vi "PostBuild.vi"(8 "error in (no error)":errorcluster, 9 "GeneratedFiles in":path[](array[path]), 10 "GeneratedDirectories in":path[](array[path]), 11 "Class in":refnum<class "Installer.lvclass">) -> (0 "error out":errorcluster, 1 "GeneratedFiles out":path[](array[path]), 2 "GeneratedDirectories out":path[](array[path]), 3 "Class out":refnum<class "Installer.lvclass">)   [LabVIEW 2020, in "Installer.lvclass"]
uses:
  <vilib>/AppBuilder/IB_Classes/Installer/Installer.lvclass
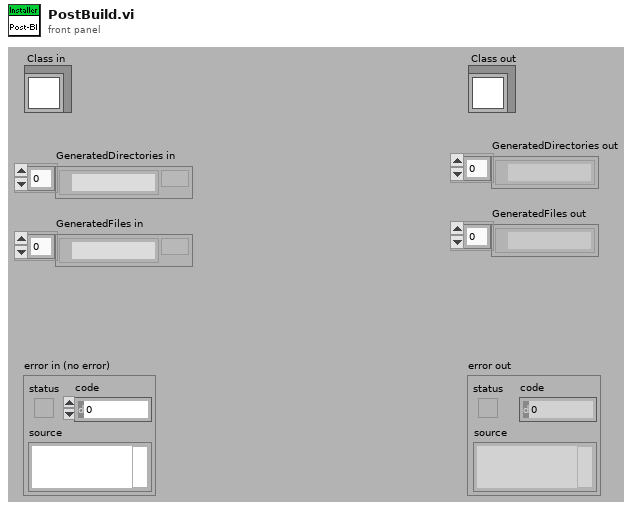
[diagram p1: front panel]
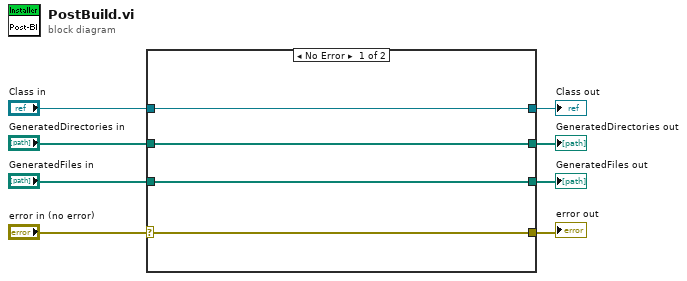
[diagram p0: block diagram]
diagram:
  n1 = case shown="No Error" "error in (no error)" {
    selector: "error in (no error)" -> [w11 w16]
    tunnel: [w11 w16] -> w7
    tunnel: [w12 w15] -> w5
    tunnel: "Class in" -> [w12 w15]
    tunnel: [w10 w14] -> w4
    tunnel: "GeneratedDirectories in" -> [w10 w14]
    tunnel: [w9 w13] -> w2
    tunnel: "GeneratedFiles in" -> [w9 w13]
    frame No Error {
    }
    frame Error {
    }
  }
  "error out" <- w7
  "Class out" <- w5
  "GeneratedDirectories out" <- w4
  "GeneratedFiles out" <- w2
